vi "Target - Async.vi"(9 "Wait (ms)":u32, 10 "Y":dbl, 11 "X":dbl) -> (3 "X + Y":dbl)   [LabVIEW 2016]
doc: "Target VI used in conjunction with the asynchronous call examples."
panel:
  in  "stop":bool
  out "Elapsed Time (s)":dbl format="%.1g"
  # "Target VI used with the asynchronous call examples."
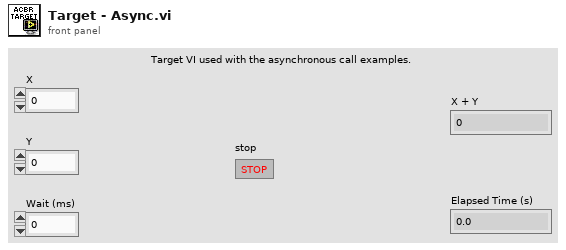
[diagram p1: front panel]
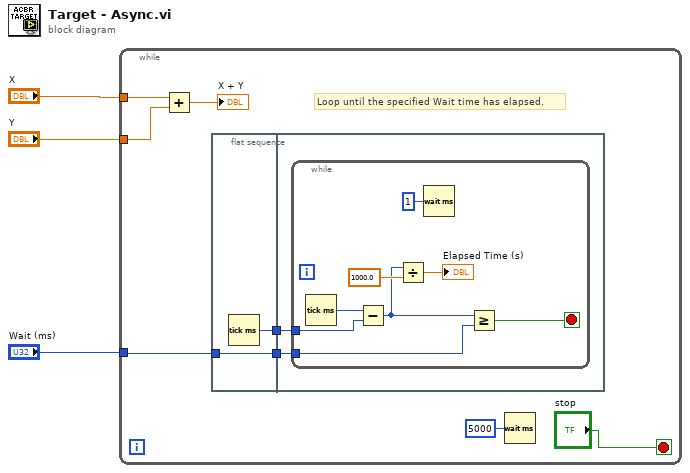
[diagram p0: block diagram]
diagram:
  n1 = while {
    tunnel: "X" -> [w9]
    tunnel: "Y" -> [w8]
    tunnel: "Wait (ms)" -> [w6]
    stop <- "stop" stop-if-true
    # "Loop until the specified Wait time has elapsed."
    n2 = Add(x=w9, y=w8) -> (x+y=→"X + Y":dbl)
    n3 = flat-sequence {
      tunnel: [w13] -> w11
      tunnel: [w12] -> w10
      tunnel: w6 -> [w12]
      tunnel: w11 -> [w15]
      tunnel: w10 -> [w14]
      frame #0 {
        n4 = Tick Count (ms)() -> (millisecond timer value=w13:u32)
      }
      frame #1 {
        n5 = while {
          tunnel: w15 -> [w21]
          tunnel: w14 -> [w19]
          stop <- w20 stop-if-true
          n6 = Tick Count (ms)() -> (millisecond timer value=w18:u32)
          n7 = Subtract(x=w18, y=w21) -> (x-y=w17:u32)
          n8 = Divide(x=w17, y=1000.0) -> (x/y=→"Elapsed Time (s)":dbl)
          n9 = Wait (ms)(milliseconds to wait=u32 1) -> ()  [unwired: 1 out]
          n10 = Greater Or Equal?(x=w17, y=w19) -> (x >= y?=w20:bool)
        }
      }
    }
    n11 = Wait (ms)(milliseconds to wait=u32 5000) -> ()  [unwired: 1 out]
  }
